vi "CheckStopping.vi"(11 "Lifetime":T1) -> (3 "Stopping":bool)   [LabVIEW 2020, in "jettl.lvlib"]
uses:
  jettl.lvlib
  Lifetime.ctl
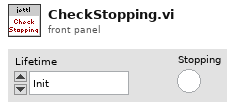
[diagram p1: front panel]
types:
  T1 = typedef "jettl.lvlib/Lifetime.ctl" = enum16{"Init", "Spawn", "Setup", "TeardownBeforeRunning", "Running", "StopCalled", "StoppingWithComponents", "StoppingNoComponents", "TeardownAfterRunning", "Stopped"}
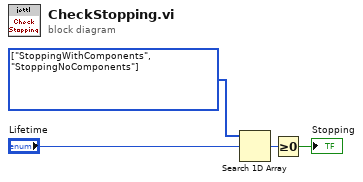
[diagram p0: block diagram]
diagram:
  w1 = T1[] [enum."StoppingWithComponents", enum."StoppingNoComponents"] items=["Init", "Spawn", "Setup", "TeardownBeforeRunning", "Running", "StopCalled", "StoppingWithComponents", "StoppingNoComponents", "TeardownAfterRunning", "Stopped"]
  n1 = Search 1D Array(1D array=w1, element="Lifetime") -> (index of element=w4:i32)  [unwired: 1 in]
  n2 = Greater Or Equal To 0?(x=w4) -> (x >= 0?=→"Stopping":bool)
